vi "Cart.vi"   [LabVIEW 2016]
uses:
  <vilib>/NXT/NXTIO Xnodes/NXTIONodeSubVIs/LEGOMoveAllMotorsDistance.vi
  <vilib>/NXT/Subs/LVHSConnector.ctl
  <vilib>/NXT/NXTIO Xnodes/NXTIOXNode/NXTIO.xnode
  <vilib>/NXT/LegoClasses/BrickReference/BrickReference.lvclass
types:
  T1 = typedef "LVHSConnector.ctl" = refnum<class "BrickReference.lvclass">
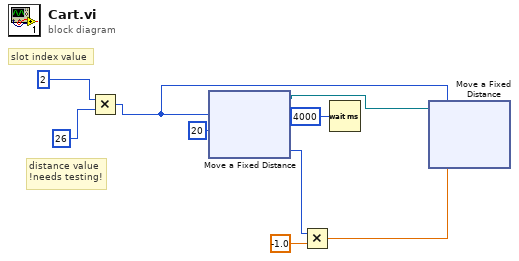
[diagram p0: block diagram]
diagram:
  w2 = i8 20 ("Speed 1")
  # "distance value\n!needs testing!"
  # "slot index value"
  n1 = Multiply(x=2, y=26) -> (x*y=w4:i32)
  n2 = xnode "Move a Fixed Distance"("Speed 1"=w2, "Distance 1"=w4) -> ("NXT/EV3"=w5:T1)  [unwired: 2 in]
  n3 = Multiply(x=w2, y=-1.0) -> (x*y=w1:dbl)
  n4 = Wait (ms)(milliseconds to wait=u32 4000) -> ()  [unwired: 1 out]
  n5 = xnode "Move a Fixed Distance"("Speed 1"=w1, "Distance 1"=w4, "NXT/EV3"=w5) -> ()  [unwired: 1 in, 1 out]
